vi "get_mag_inputs.vi"(8 "error in (no error)":errorcluster, 11 "magnetometer in":refnum<class "magnetometer.lvclass">) -> (0 "error out":errorcluster, 2 "mag inputs":T1, 3 "magnetometer out":refnum<class "magnetometer.lvclass">)   [LabVIEW 2015, in "magnetometer.lvclass"]
uses:
  magnetometer.lvclass
  magnetometer.lvclass/magnetometer.ctl
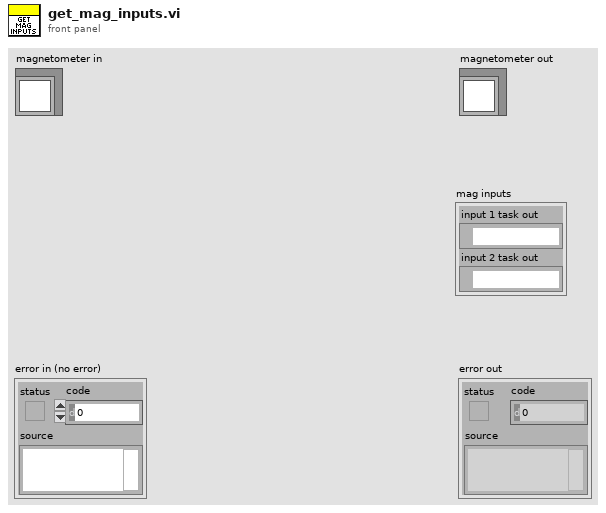
[diagram p1: front panel]
types:
  T1 = cluster{"input 1 task out":refnum<k21>, "input 2 task out":refnum<k21>}
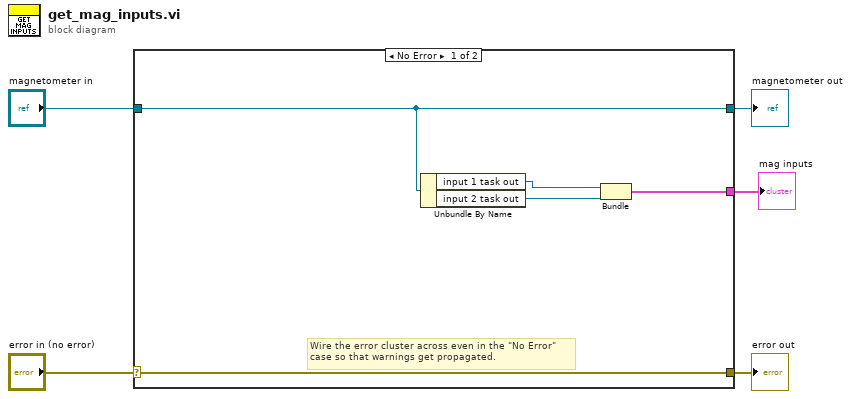
[diagram p0: block diagram]
diagram:
  n1 = case shown="No Error" "error in (no error)" {
    selector: "error in (no error)" -> [w10 w12]
    tunnel: [w10 w12] -> w4
    tunnel: [w9 w11] -> w2
    tunnel: "magnetometer in" -> [w9 w11]
    tunnel: [w6 _] -> w1
    frame No Error {
      # "Wire the error cluster across even in the \"No Error\"\ncase so that warnings get propagated."
      n2 = Unbundle By Name(w9) -> ("input 1 task out"=w8:refnum<k21>, "input 2 task out"=w7:refnum<k21>)
      n3 = Bundle("input 1 task out"=w8, "input 2 task out"=w7) -> (w6:T1)  [unwired: 1 in]
    }
    frame Error {
    }
  }
  "error out" <- w4
  "magnetometer out" <- w2
  "mag inputs" <- w1
